vi "PLC_OP30_Write.vi"(8 "error in (no error)":errorcluster, 10 "FIRST CALL AFTER ERROR":bool, 11 "S7 Connection in":T1) -> (0 "error out":errorcluster, 3 "S7 Connection out":T1)   [LabVIEW 2017]
uses:
  <vilib>/DATA AHEAD/SP7/typedefs/S7 Connection.ctl
  <vilib>/DATA AHEAD/SP7/typedefs/PLC Type.ctl
  5bdceb99-9d6b-4556-ab7e-9eda66c057e4.vi
  Global/DATA LOG.vi
  <vilib>/DATA AHEAD/SP7/functions/write/write Dint array.vi
  Global/Global 1.vi
  <vilib>/DATA AHEAD/SP7/functions/write/writeString.vi
  <vilib>/DATA AHEAD/SP7/SP7.lvlib
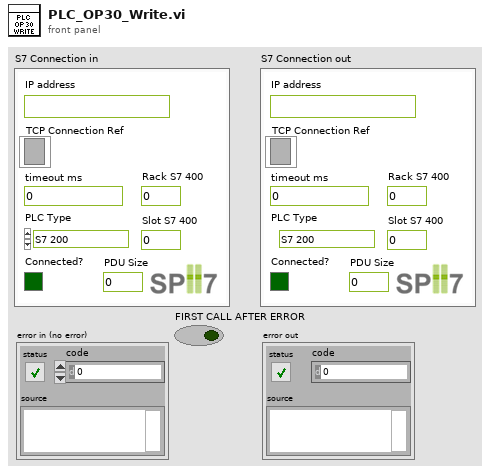
[diagram p1: front panel]
types:
  T1 = typedef "SP7.lvlib/S7 Connection.ctl" = cluster{"TCP Connection Ref":refnum<k5>, "IP address":string, "timeout ms":i32, "Connected?":bool, "PLC Type":T2, "Rack S7 400":u8, "Slot S7 400":u8, "PDU Size":u16, "connection semaphore":T3}
  T2 = typedef "SP7.lvlib/PLC Type.ctl" = enum16{"S7 200", "S7 300/400", "S7 1200", "S7 1500", "LOGO!8"}
  T3 = typedef "Semaphore RefNum" = refnum<k1>
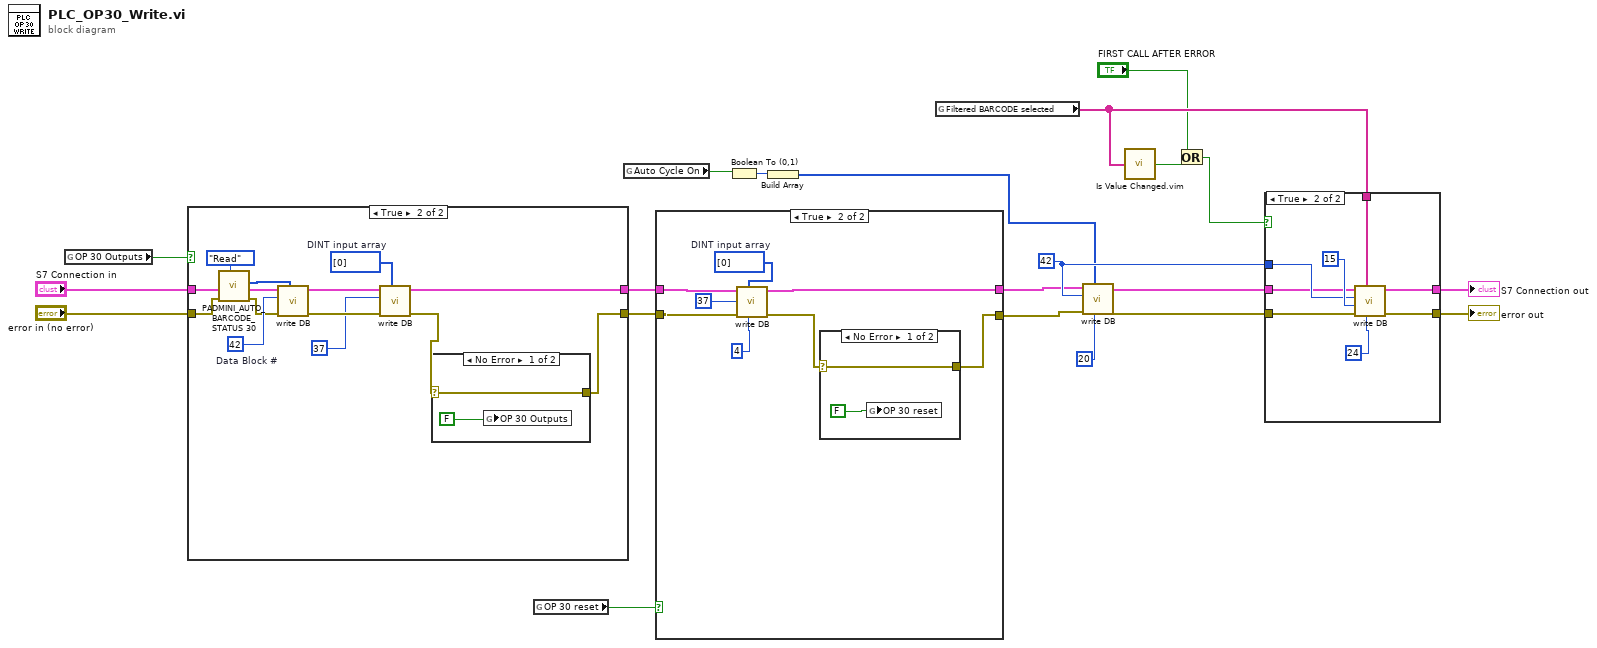
[diagram p0: block diagram]
diagram:
  w21 = u16 42 ("Data Block #")
  n1 = global read "DATA LOG.vi" "OP 30 Outputs"() -> (w10:bool)
  n2 = case shown="True" w10 {
    tunnel: "S7 Connection in" -> [w22 w35]
    tunnel: [w23 w24] -> w11
    tunnel: [w22 w29] -> w12
    tunnel: "error in (no error)" -> [w23 w32]
    frame False {
    }
    frame True {
      w27 = i32[] [0]  # DINT input array
      w36 = u16 42  # Data Block #
      n3 = call "PADMINI_AUTO_BARCODE_STATUS 30.vi"("Enum"=enum16{"Read", "Write"}."Read", "error in (no error)"=w32) -> ("error out"=w31:errorcluster, "O/P"=w33:i32[])  [unwired: 8 in]
      n4 = call-poly <vilib>:"write DB.vi"("DINT input array"=w33, "error in (no error)"=w31, "Data Block #"=w36, "S7 Connection in"=w35) -> ("error out"=w30:errorcluster, "S7 Connection out"=w28:T1)  [unwired: 4 in, 2 out]
      n5 = call-poly <vilib>:"write DB.vi"("DINT input array"=w27, "error in (no error)"=w30, "Data Block #"=u16 37, "S7 Connection in"=w28) -> ("error out"=w25:errorcluster, "S7 Connection out"=w29:T1)  [unwired: 4 in, 2 out]
      n6 = case shown="No Error" w25 {
        selector: w25 -> [w37 w39]
        tunnel: [w37 w39] -> w24
        frame No Error {
          n7 = global write "DATA LOG.vi" "OP 30 Outputs"(FALSE) -> ()
        }
        frame Error {
        }
      }
    }
  }
  n8 = global read "DATA LOG.vi" "OP 30 reset"() -> (w13:bool)
  n9 = global read "DATA LOG.vi" "Auto Cycle On"() -> (w7:bool)
  n10 = case shown="True" w13 {
    tunnel: w11 -> [w40 w49]
    tunnel: [w40 w42] -> w18
    tunnel: w12 -> [w41 w48]
    tunnel: [w41 w47] -> w16
    frame False {
    }
    frame True {
      w46 = i32[] [0]  # DINT input array
      n11 = call-poly <vilib>:"write DB.vi"("Item offset [byte]"=u16 4 ("Data Block #"), "DINT input array"=w46, "error in (no error)"=w49, "Data Block #"=u16 37, "S7 Connection in"=w48) -> ("error out"=w43:errorcluster, "S7 Connection out"=w47:T1)  [unwired: 3 in, 2 out]
      n12 = case shown="No Error" w43 {
        selector: w43 -> [w50 w52]
        tunnel: [w50 w52] -> w42
        frame No Error {
          n13 = global write "DATA LOG.vi" "OP 30 reset"(FALSE) -> ()
        }
        frame Error {
        }
      }
    }
  }
  n14 = Boolean To (0,1)(Boolean=w7) -> (0, 1=w6:i16)
  n15 = Build Array(w6) -> (w5:i16[])
  n16 = global read "Global 1.vi" "Filtered BARCODE selected"() -> (w4:string[])
  n17 = call-poly <vilib>:"write DB.vi"("Item offset [byte]"=u32 20, "DINT input array"=w5, "error in (no error)"=w18, "Data Block #"=w21, "S7 Connection in"=w16) -> ("error out"=w15:errorcluster, "S7 Connection out"=w14:T1)  [unwired: 3 in, 2 out]
  n18 = call "Is Value Changed.vim"("value"=w4) -> ("changed or first call?"=w3:bool)
  n19 = Or(x="FIRST CALL AFTER ERROR", y=w3) -> (x .or. y?=w2:bool)
  n20 = case shown="True" w2 {
    tunnel: w4 -> [_ w62]
    tunnel: w21 -> [_ w59]
    tunnel: [w53 w58] -> w19
    tunnel: [w54 w57] -> w17
    tunnel: w15 -> [w53 w56]
    tunnel: w14 -> [w54 w55]
    frame False {
    }
    frame True {
      n21 = call-poly <vilib>:"write DB.vi"("Item offset [byte]"=u32 24, "Input STRINGS"=w62, "error in (no error)"=w56, "String length reserved in DB (default=254)"=u16 15, "Data Block #"=w59, "S7 Connection in"=w55) -> ("error out"=w58:errorcluster, "S7 Connection out"=w57:T1)  [unwired: 2 in, 2 out]
    }
  }
  "error out" <- w19
  "S7 Connection out" <- w17
